vi "niWLAN - OPPO - 80211abgnGeneration(ref)_bc.vi"(0 "Rx Measurements Settings":T2 {"DSSS Data Rate (Mbps)" items=["1", "2", "5.5 CCK", "5.5 PBCC", "11 CCK", "11 PBCC", "22", "33"]; "OFDM Data Rate (Mbps)" items=["6", "9", "12", "18", "24", "36", "48", "54"]; "80211n PLCP Frame Format" items=["Mixed Format", "Greenfield Format"]; "Standard" items=["80211A/G/J/P OFDM", "80211B/G DSSS", "80211G DSSSOFDM", "80211N MIMOOFDM", "80211AC MIMOOFDM"]}, 5 "Without ACK ?":bool, 7 "Address String":string="00:90:4C:C5:12:38", 11 "error in":errorcluster) -> (4 "Cluster":T1, 15 "error out":errorcluster)   [LabVIEW 2012]
uses:
  TV/RW/Includes/WLAN - TV - RW - INC - Rx_PER_Wfm_Settings.ctl
  <vilib>/RF Toolkits/WLAN/generation/controls/wlanG version control.ctl
  <vilib>/RF Toolkits/WLAN/generation/niWLANG Create Multiple Channel Waveform (IQ Complex Cluster).vi
  <vilib>/RF Toolkits/WLAN/generation/niWLANG Create Single Channel Waveform (IQ Complex Cluster).vi
  <resource>/objmgr/niWLANGeneration.rc
panel:
  out "32bit integer":i32
  out "1/x":dbl
  in  "Boolean":bool
  in  "Idle Time (With Ack)":dbl
  in  "file path":path
  # "Hardware Configuration"
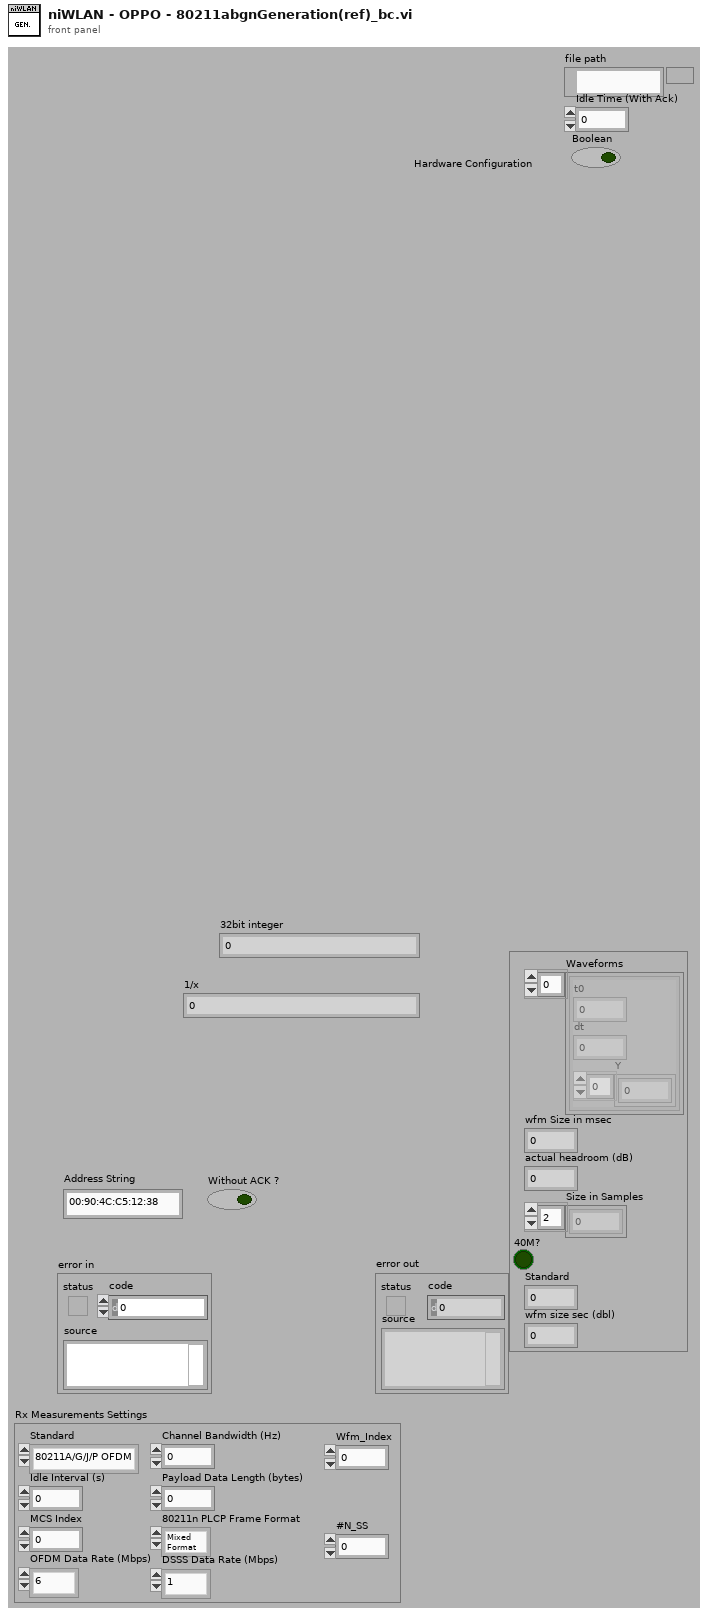
[diagram p1: front panel]
types:
  T1 = cluster{"Waveforms":cluster{"t0":dbl, "dt":dbl, "Y":cdb[]}[], "wfm Size in msec":i32, "actual headroom (dB)":dbl, "Size in Samples":i32[], "40M?":bool, "Standard ":i32, "wfm size sec (dbl)":dbl}
  T2 = typedef "WLAN - TV - RW - INC - Rx_PER_Wfm_Settings.ctl" = cluster{"Standard":i32, "Channel Bandwidth (Hz)":dbl, "Idle Interval (s)":dbl, "MCS Index":i32, "80211n PLCP Frame Format":i32, "Payload Data Length (bytes)":i32, "OFDM Data Rate (Mbps)":i32, "DSSS Data Rate (Mbps)":i32, "Wfm_Index":i32, "#N_SS":i32}
  T3 = typedef "wlanG version control.ctl" = i32
  T4 = typedef "wlanv1_generation refnum.ctl" = refnum<k20>
  T5 = typedef "wlanv1_Generation Refnum.ctl" = refnum<k20>
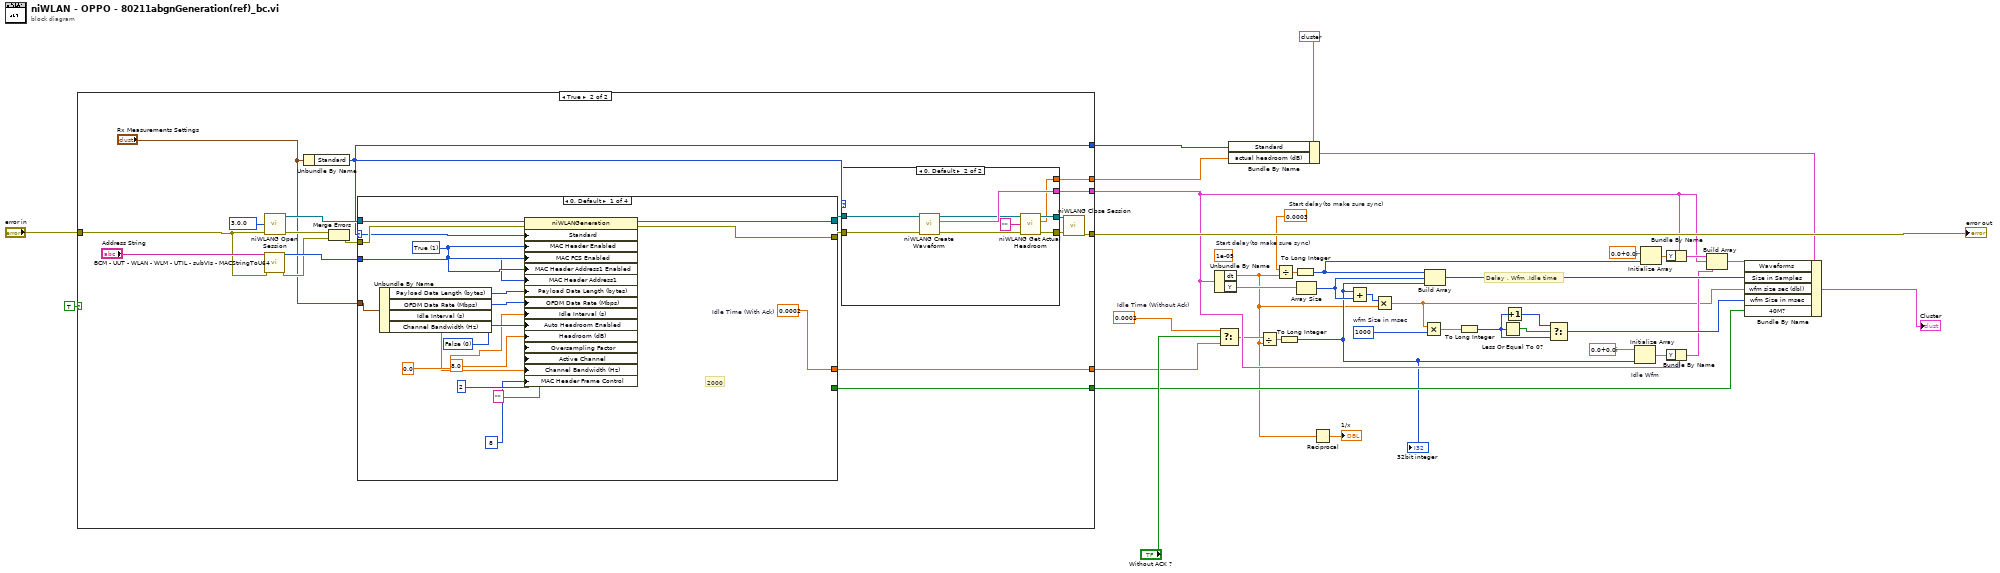
[diagram p0: block diagram]
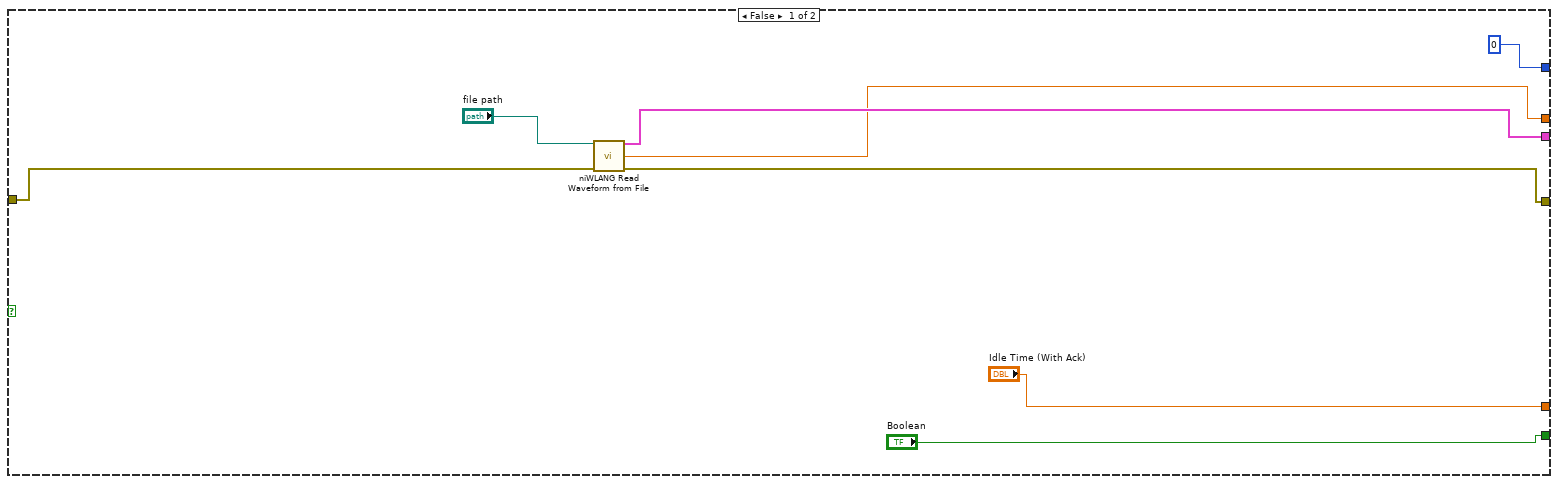
[diagram p2: hidden frame]
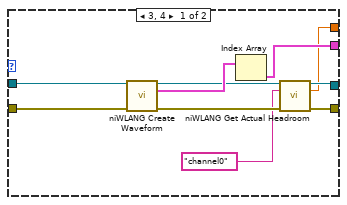
[diagram p3: hidden frame]
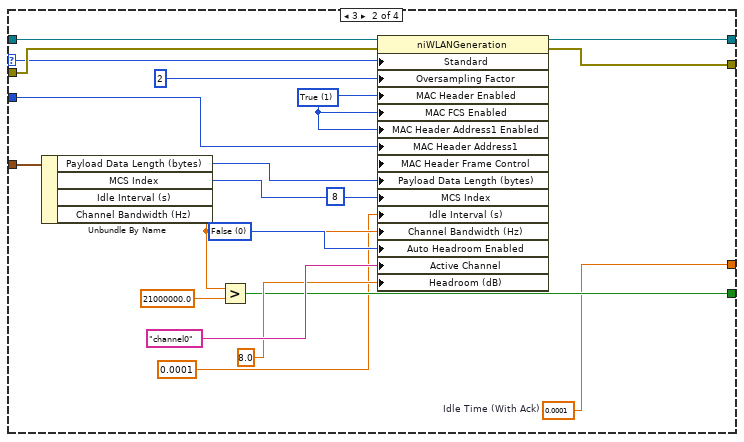
[diagram p4: hidden frame]
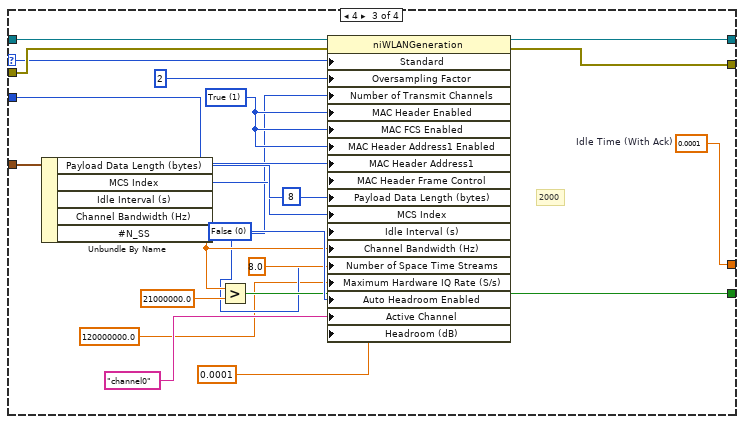
[diagram p5: hidden frame]
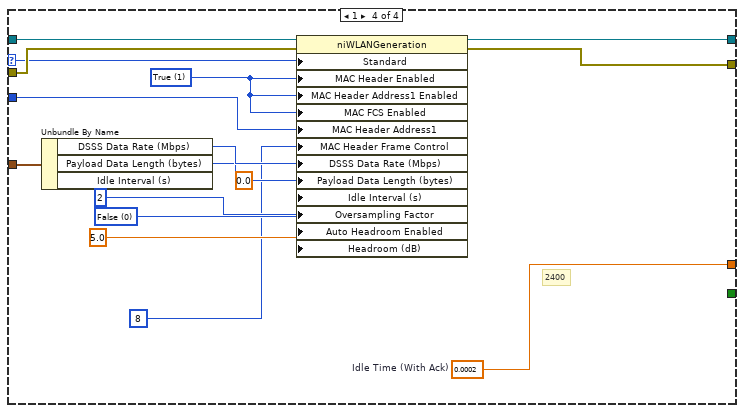
[diagram p6: hidden frame]
diagram:
  w5 = 0.0003  # Start delay(to make sure sync)
  (unwired) 1e-05  # Start delay(to make sure sync)
  w8 = 0.0002  # Idle Time (Without Ack)
  w17 = 1000  # wfm Size in msec
  # "Delay , Wfm ,Idle time"
  n1 = case shown="True" TRUE {
    tunnel: [w44 w65] -> w39
    tunnel: "error in" -> [w41 w64]
    tunnel: ["Boolean" w53] -> w25
    tunnel: [w46 w52] -> w18
    tunnel: [0 ("Standard") w51] -> w12
    tunnel: [w45 w50] -> w10
    tunnel: ["Idle Time (With Ack)" w49] -> w6
    frame False {
      n2 = call <vilib>:"niWLANG Read Waveform from File.vi"("file path"="file path", "error in"=w41) -> ("waveform"=w46:cluster{"t0":dbl, "dt":dbl, "Y":cdb[]}, "headroom (dB)"=w45:dbl, "error out"=w44:errorcluster)  [unwired: 9 in, 2 out]
    }
    frame True {
      w61 = T3 30000 items=["1.0.0"=10000, "2.0.0"=20000, "3.0.0"=30000] ("toolkit compatibility version")
      n3 = call "BCM - UUT - WLAN - WLM - UTIL - subVIs - MACStringToU64.vi"("Address String"="Address String", "error in"=w64) -> ("Address U64"=w63:u64, "error out"=w59:errorcluster)  [unwired: 12 in]
      n4 = call <vilib>:"niWLANG Open Session.vi"("toolkit compatibility version"=w61, "error in"=w64) -> ("niwlan generation session"=w62:T4, "error out"=w60:errorcluster)  [unwired: 11 in, 1 out]
      n5 = Unbundle By Name("Rx Measurements Settings") -> ("Standard"=w51:i32)
      n6 = Merge Errors(w60, w59) -> (w58:errorcluster)
      n7 = case shown="0, Default" w51 {
        selector: w51 -> [w98 w118 w140 w158]
        tunnel: w62 -> [w103 w122 w144 w161]
        tunnel: w58 -> [w102 w119 w141 w160]
        tunnel: [w101 w121 w143 w159] -> w55
        tunnel: [w100 w120 w142 w149] -> w54
        tunnel: w63 -> [w93 w111 w133 w154]
        tunnel: "Rx Measurements Settings" -> [w91 w115 w137 w150]
        tunnel: [_ w107 w129 _] -> w53
        tunnel: [w89 w105 w127 w147] -> w49
        frame 0, Default {
          w89 = 0.0002  # Idle Time (With Ack)
          w96 = 0 items=["False", "True"] ("Auto Headroom Enabled")
          w99 = 1 items=["False", "True"] ("MAC Header Enabled")
          # "2000"
          n8 = Unbundle By Name(w91) -> ("Payload Data Length (bytes)"=w94:i32, "OFDM Data Rate (Mbps)"=w97:i32, "Channel Bandwidth (Hz)"=w87:dbl)  [unwired: 1 out]
          n9 = property class="niWLANGeneration"(reference=w103, error in=w102, "Standard"=w98, "MAC Header Enabled"=w99, "MAC FCS Enabled"=w99, "MAC Header Address1 Enabled"=w99, "MAC Header Address1"=w93, "Payload Data Length (bytes)"=w94, "OFDM Data Rate (Mbps)"=w97, "Idle Interval (s)"=0.0, "Auto Headroom Enabled"=w96, "Headroom (dB)"=8.0, "Oversampling Factor"=2, "Active Channel"="", "Channel Bandwidth (Hz)"=w87, "MAC Header Frame Control"=8) -> (reference out=w101:T4, error out=w100:errorcluster)
        }
        frame 3 {
          w105 = 0.0001  # Idle Time (With Ack)
          w114 = 0 items=["False", "True"] ("Auto Headroom Enabled")
          w123 = 1 items=["False", "True"] ("MAC Header Enabled")
          n10 = Unbundle By Name(w115) -> ("Payload Data Length (bytes)"=w117:i32, "MCS Index"=w116:i32, "Channel Bandwidth (Hz)"=w110:dbl)  [unwired: 1 out]
          n11 = Greater?(x=w110, y=21000000.0) -> (0:w107:bool)
          n12 = property class="niWLANGeneration"(reference=w122, error in=w119, "Standard"=w118, "Oversampling Factor"=2, "MAC Header Enabled"=w123, "MAC FCS Enabled"=w123, "MAC Header Address1 Enabled"=w123, "MAC Header Address1"=w111, "MAC Header Frame Control"=8, "Payload Data Length (bytes)"=w117, "MCS Index"=w116, "Idle Interval (s)"=0.0001, "Channel Bandwidth (Hz)"=w110, "Auto Headroom Enabled"=w114, "Active Channel"="channel0", "Headroom (dB)"=8.0) -> (reference out=w121:T4, error out=w120:errorcluster)
        }
        frame 4 {
          w127 = 0.0001  # Idle Time (With Ack)
          w136 = 0 items=["False", "True"] ("Auto Headroom Enabled")
          w145 = 1 items=["False", "True"] ("MAC Header Enabled")
          # "2000"
          n13 = Unbundle By Name(w137) -> ("Payload Data Length (bytes)"=w139:i32, "MCS Index"=w138:i32, "Channel Bandwidth (Hz)"=w132:dbl, "#N_SS"=w125:i32)  [unwired: 1 out]
          n14 = Greater?(x=w132, y=21000000.0) -> (0:w129:bool)
          n15 = property class="niWLANGeneration"(reference=w144, error in=w141, "Standard"=w140, "Oversampling Factor"=2, "Number of Transmit Channels"=w125, "MAC Header Enabled"=w145, "MAC FCS Enabled"=w145, "MAC Header Address1 Enabled"=w145, "MAC Header Address1"=w133, "MAC Header Frame Control"=8, "Payload Data Length (bytes)"=w139, "MCS Index"=w138, "Idle Interval (s)"=0.0001, "Channel Bandwidth (Hz)"=w132, "Number of Space Time Streams"=w125, "Maximum Hardware IQ Rate (S/s)"=120000000.0, "Auto Headroom Enabled"=w136, "Active Channel"="channel0", "Headroom (dB)"=8.0) -> (reference out=w143:T4, error out=w142:errorcluster)
        }
        frame 1 {
          w147 = 0.0002  # Idle Time (With Ack)
          w152 = 0 items=["False", "True"] ("Auto Headroom Enabled")
          w157 = 1 items=["False", "True"] ("OFDM Demod Enabled")
          # "2400"
          n16 = Unbundle By Name(w150) -> ("DSSS Data Rate (Mbps)"=w156:i32, "Payload Data Length (bytes)"=w155:i32)  [unwired: 1 out]
          n17 = property class="niWLANGeneration"(reference=w161, error in=w160, "Standard"=w158, "MAC Header Enabled"=w157, "MAC Header Address1 Enabled"=w157, "MAC FCS Enabled"=w157, "MAC Header Address1"=w154, "MAC Header Frame Control"=8, "DSSS Data Rate (Mbps)"=w156, "Payload Data Length (bytes)"=w155, "Idle Interval (s)"=0.0, "Oversampling Factor"=2, "Auto Headroom Enabled"=w152, "Headroom (dB)"=5.0) -> (reference out=w159:T4, error out=w149:errorcluster)
        }
      }
      n18 = case shown="0, Default" w51 {
        tunnel: [w71 w81] -> w56
        tunnel: w55 -> [w75 w85]
        tunnel: w54 -> [w76 w84]
        tunnel: [w69 w80] -> w57
        tunnel: [w73 w83] -> w52
        tunnel: [w67 w78] -> w50
        frame 3, 4 {
          n19 = call-poly <vilib>:"niWLANG Create Waveform.vi"("niwlan generation session"=w75, "error in"=w76) -> ("niwlan generation session out"=w72:T4, "output waveform"=w74:cluster{"t0":dbl, "dt":dbl, "Y":cdb[]}[], "error out"=w70:errorcluster)  [unwired: 10 in, 1 out]
          n20 = Index Array(array=w74) -> (element=w73:cluster{"t0":dbl, "dt":dbl, "Y":cdb[]})  [unwired: 1 in]
          n21 = call <vilib>:"niWLANG Get Actual Headroom.vi"("niwlan generation session"=w72, "active channel"="channel0", "error in"=w70) -> ("niwlan generation session out"=w71:T5, "actual headroom (dB)"=w67:dbl, "error out"=w69:errorcluster)  [unwired: 10 in]
        }
        frame 0, Default {
          n22 = call-poly <vilib>:"niWLANG Create Waveform.vi"("niwlan generation session"=w85, "error in"=w84) -> ("niwlan generation session out"=w82:T4, "output waveform"=w83:cluster{"t0":dbl, "dt":dbl, "Y":cdb[]}, "error out"=w79:errorcluster)  [unwired: 10 in, 1 out]
          n23 = call <vilib>:"niWLANG Get Actual Headroom.vi"("niwlan generation session"=w82, "active channel"="", "error in"=w79) -> ("niwlan generation session out"=w81:T5, "actual headroom (dB)"=w78:dbl, "error out"=w80:errorcluster)  [unwired: 10 in]
        }
      }
      n24 = call <vilib>:"niWLANG Close Session.vi"("niwlan generation session"=w56, "error in"=w57) -> ("error out"=w65:errorcluster)  [unwired: 13 in]
    }
  }
  "error out" <- w39
  n25 = Unbundle By Name(w18) -> ("dt"=w2:dbl, "Y"=w13:cdb[])
  n26 = Select(t=w8, s="Without ACK ?", f=w6) -> (s? t:f=w7:dbl)
  n27 = Bundle By Name(cluster=T1 {"Waveforms"=[{"t0"=0.0, "dt"=1.25e-08, "Y"=array[800 elements]}, {"t0"=0.0, "dt"=1.25e-08, "Y"=array[85448 elements]}], "wfm Size in msec"=1, "actual headroom (dB)"=0.0, "Size in Samples"=[10000000, 0], "40M?"=TRUE, "Standard "=3, "wfm size sec (dbl)"=0.0} ("Cluster"), "Standard"=w12, "actual headroom (dB)"=w10) -> (w11:T1)
  n28 = Divide(x=w7, y=w2) -> (x/y=w20:dbl)
  n29 = Divide(x=w5, y=w2) -> (x/y=w32:dbl)
  n30 = To Long Integer(number=w20) -> (32bit integer=w9:i32)
  "32bit integer" <- w9
  n31 = To Long Integer(number=w32) -> (32bit integer=w31:i32)
  n32 = Array Size(array=w13) -> (size(s)=w21:i32)
  n33 = Reciprocal(x=w2) -> (1/x=→"1/x":dbl)
  n34 = Add(x=w9, y=w21) -> (x+y=w19:i32)
  n35 = Multiply(x=w19, y=w2) -> (x*y=w15:dbl)
  n36 = Multiply(x=w15, y=w17) -> (x*y=w16:dbl)
  n37 = Build Array(w31, w21, w9) -> (w27:i32[])
  n38 = To Long Integer(number=w16) -> (32bit integer=w34:i32)
  n39 = Less Or Equal To 0?(x=w34) -> (x <= 0?=w35:bool)
  n40 = Increment(x=w34) -> (x+1=w33:i32)
  n41 = Select(t=w33, s=w35, f=w34) -> (s? t:f=w26:i32)
  n42 = Initialize Array "Idle Wfm"(cdb 0.0+0.0i ("element"), w9) -> (w23:cdb[])
  n43 = Initialize Array(cdb 0.0+0.0i ("element"), w31) -> (w30:cdb[])
  n44 = Bundle By Name(cluster=w18, "Y"=w30) -> (w29:cluster{"t0":dbl, "dt":dbl, "Y":cdb[]})
  n45 = Bundle By Name(cluster=w18, "Y"=w23) -> (w22:cluster{"t0":dbl, "dt":dbl, "Y":cdb[]})
  n46 = Build Array(w29, w18, w22) -> (w28:cluster{"t0":dbl, "dt":dbl, "Y":cdb[]}[])
  n47 = Bundle By Name(cluster=w11, "Waveforms"=w28, "Size in Samples"=w27, "wfm size sec (dbl)"=w15, "wfm Size in msec"=w26, "40M?"=w25) -> (→"Cluster":T1)
